vi "5.10 Generate Behavior.vi"(0 "Numeric":dbl, 1 "Location of Camera":dbl[](array[numeric]), 2 "Rotation of Camera":dbl[][](array[numeric]), 3 "Numeric 2":dbl, 4 "Line Def":T1) -> (5 "Drive Angles":dbl[](array[numeric]), 6 "Array":dbl[](array[numeric]))   [LabVIEW 2011]
uses:
  6-OCU Neurons/6.10 Occipital Neurons/6.10.1 LineDef.ctl
  <vilib>/Analysis/Matrix/Numeric/Conversions/Array To Matrix - RA.vi
  <vilib>/Analysis/Matrix/Numeric/Conversions/Array To Matrix - RA2.vi
  <vilib>/Analysis/Matrix/NI_Matrix.lvlib
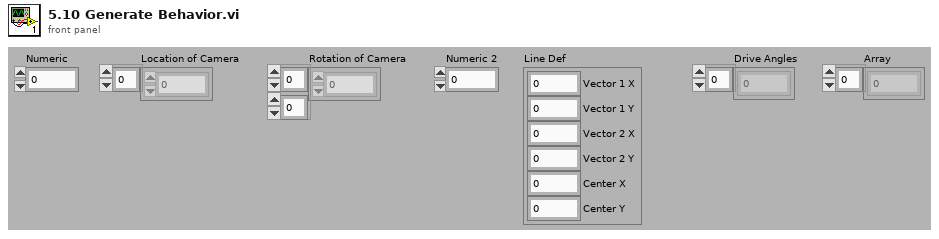
[diagram p1: front panel]
types:
  T1 = typedef "6.10.1 LineDef.ctl" = cluster{"Vector 1 X":dbl, "Vector 1 Y":dbl, "Vector 2 X":dbl, "Vector 2 Y":dbl, "Center X":dbl, "Center Y":dbl}
  T2 = typedef "NI_Matrix.lvlib/RealMatrix.ctl" = dbl[][]
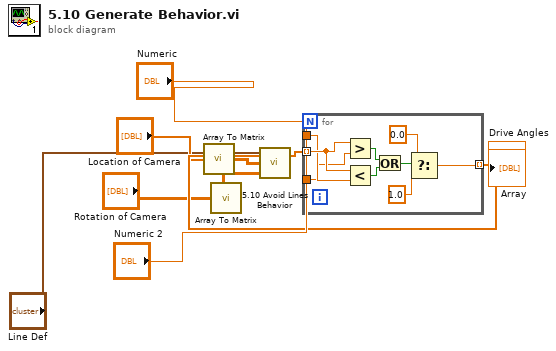
[diagram p0: block diagram]
diagram:
  n1 = call-poly <vilib>:"Array To Matrix.vi"("Real 1D Array"="Location of Camera") -> ("Real Matrix (Column Vector)"=w4:T2)
  n2 = call-poly <vilib>:"Array To Matrix.vi"("Real 2D Array"="Rotation of Camera") -> ("Real Matrix"=w5:T2)
  n3 = call "5.10 Avoid Lines Behavior.vi"("Rotation of Camera"=w5, "Location of Camera"=w4, "Line Def"="Line Def") -> ("Drive Angles"=w6:dbl[])  [unwired: 1 out]
  "Drive Angles" <- w6
  n4 = for {
    tunnel: w6 -> [w18] mode=indexing
    tunnel: "Numeric 2" -> [w17]
    tunnel: "Numeric" -> [w16]
    tunnel: [w10] -> w9 mode=indexing
    n5 = Greater?(x=w18, y=w16) -> (0:w14:bool)
    n6 = Less?(x=w18, y=w17) -> (x < y?=w15:bool)
    n7 = Or(x=w14, y=w15) -> (x .or. y?=w13:bool)
    n8 = Select(t=0.0, s=w13, f=1.0) -> (s? t:f=w10:dbl)
  }
  "Array" <- w9
